vi "gyro_binary_get_time_info.vi"(8 "error in":errorcluster, 10 "all in one package in":T1={"measurement data"={"number of samples per axis"=0, "timestamp array"=[], "offset array"=[], "x, y, z axis data"=[], "magnitude of acceleartion vectors"={"t0"=timestamp(0 s since 1904-01-01), "dt"=1.0, "Y"=[]}, "statistics"={"mean of x axis acceleration"=0.0, "standard devation \nof x axis acceleration"=0.0, "mean of y axis acceleration"=0.0, "standard devation \nof y axis acceleration"=0.0, "mean of z axis acceleration"=0.0, "standard devation \nof z axis acceleration"=0.0, "mean of magnitude\n of acceleration"=0.0, "standard devation \nof magnitude of acceleration"=0.0}, "voltage"={"t0"=timestamp(0 s since 1904-01-01), "dt"=1.0, "Y"=[]}}, "actigraph settings"={"# Pages"=0, "ODR"=0, "xlRange"=0, "gyroRange"=0, "id"=0, "Samplig Freq [Hz]"=0.0, "xlRange in g"=0.0, "gyroRange in dps"=0.0}, "memory structure"={"length of metadata [byte]"=5, "length of page [byte]"=2048, "length of measurement \ndata on page [byte]"=2028, "length of dataset [byte]"=6}, "time informations"={"starting time"=timestamp(0 s since 1904-01-01), "ending time"=timestamp(0 s since 1904-01-01), "dt[s]"=0.0, "sampling rate [Hz]"=0.0, "length"=0.0}} {"time informations"."length" format="%<%H:%M:%S%3u>t"; "actigraph settings"."id" format="%02d"; "actigraph settings"."xlRange" format="%02x"; "actigraph settings"."ODR" format="%02x"}, 11 "pages":u8[](array[numeric])) -> (0 "error out":errorcluster, 2 "all in one package out":T1={"measurement data"={"number of samples per axis"=0, "timestamp array"=[], "offset array"=[], "x, y, z axis data"=[], "magnitude of acceleartion vectors"={"t0"=timestamp(0 s since 1904-01-01), "dt"=1.0, "Y"=[]}, "statistics"={"mean of x axis acceleration"=0.0, "standard devation \nof x axis acceleration"=0.0, "mean of y axis acceleration"=0.0, "standard devation \nof y axis acceleration"=0.0, "mean of z axis acceleration"=0.0, "standard devation \nof z axis acceleration"=0.0, "mean of magnitude\n of acceleration"=0.0, "standard devation \nof magnitude of acceleration"=0.0}, "voltage"={"t0"=timestamp(0 s since 1904-01-01), "dt"=1.0, "Y"=[]}}, "actigraph settings"={"# Pages"=0, "ODR"=0, "xlRange"=0, "gyroRange"=0, "id"=0, "Samplig Freq [Hz]"=0.0, "xlRange in g"=0.0, "gyroRange in dps"=0.0}, "memory structure"={"length of metadata [byte]"=5, "length of page [byte]"=2048, "length of measurement \ndata on page [byte]"=2028, "length of dataset [byte]"=6}, "time informations"={"starting time"=timestamp(0 s since 1904-01-01), "ending time"=timestamp(0 s since 1904-01-01), "dt[s]"=0.0, "sampling rate [Hz]"=0.0, "length"=0.0}} {"time informations"."length" format="%<%H:%M:%S%3u>t"; "actigraph settings"."id" format="%02d"; "actigraph settings"."xlRange" format="%02x"; "actigraph settings"."ODR" format="%02x"}, 3 "pages excluding first and last page":u8[](array[numeric]))   [LabVIEW 2019]
uses:
  Controls/gyro_control_all_in_one_package.ctl
  Controls/gyro_control_measurement_data.ctl
  Controls/gyro_control_measurement_settings.ctl
  Controls/gyro_control_memory_structure.ctl
  Controls/gyro_control_time_informations.ctl
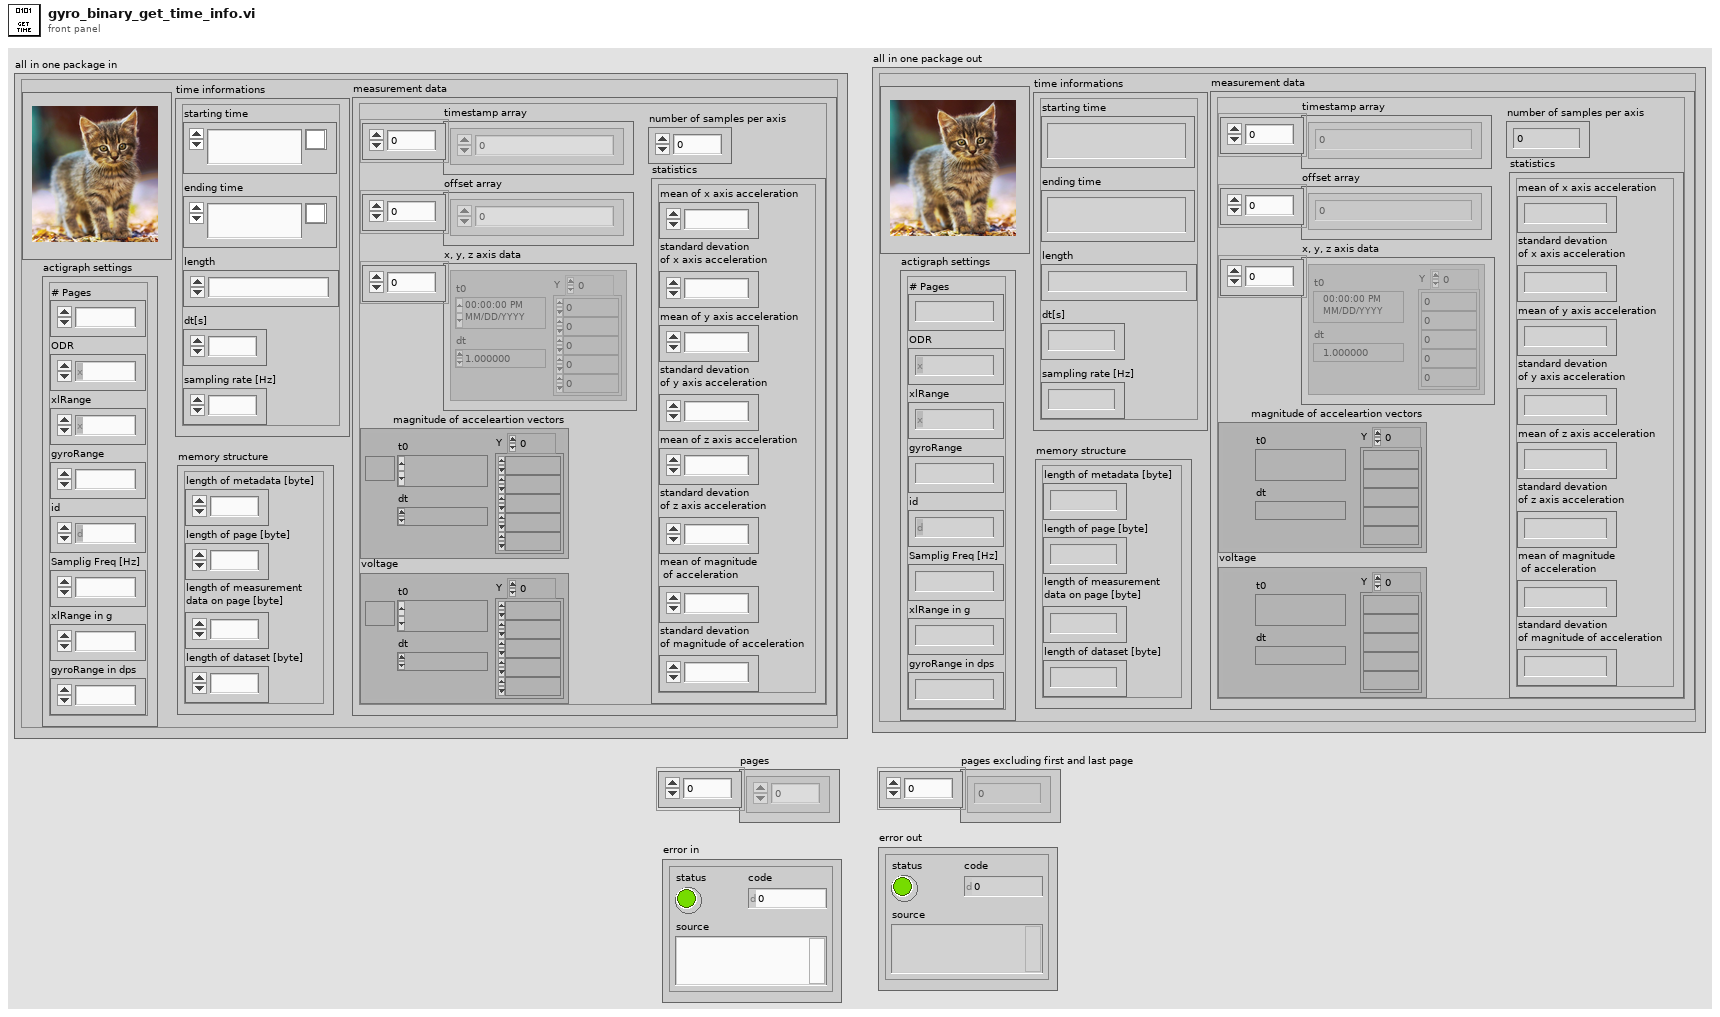
[diagram p1: front panel]
types:
  T1 = typedef "gyro_control_all_in_one_package.ctl" = cluster{"measurement data":T2, "actigraph settings":T3, "memory structure":T4, "time informations":T5}
  T2 = typedef "gyro_control_measurement_data.ctl" = cluster{"number of samples per axis":i32, "timestamp array":dbl[], "offset array":dbl[], "x, y, z axis data":waveform(dbl)[], "magnitude of acceleartion vectors":waveform(dbl), "statistics":cluster{"mean of x axis acceleration":dbl, "standard devation \nof x axis acceleration":dbl, "mean of y axis acceleration":dbl, "standard devation \nof y axis acceleration":dbl, "mean of z axis acceleration":dbl, "standard devation \nof z axis acceleration":dbl, "mean of magnitude\n of acceleration":dbl, "standard devation \nof magnitude of acceleration":dbl}, "voltage":waveform(dbl)}
  T3 = typedef "gyro_control_measurement_settings.ctl" = cluster{"# Pages":i32, "ODR":u8, "xlRange":u8, "gyroRange":u8, "id":u8, "Samplig Freq [Hz]":dbl, "xlRange in g":dbl, "gyroRange in dps":dbl}
  T4 = typedef "gyro_control_memory_structure.ctl" = cluster{"length of metadata [byte]":i32, "length of page [byte]":i32, "length of measurement \ndata on page [byte]":i32, "length of dataset [byte]":i32}
  T5 = typedef "gyro_control_time_informations.ctl" = cluster{"starting time":timestamp, "ending time":timestamp, "dt[s]":dbl, "sampling rate [Hz]":dbl, "length":dbl}
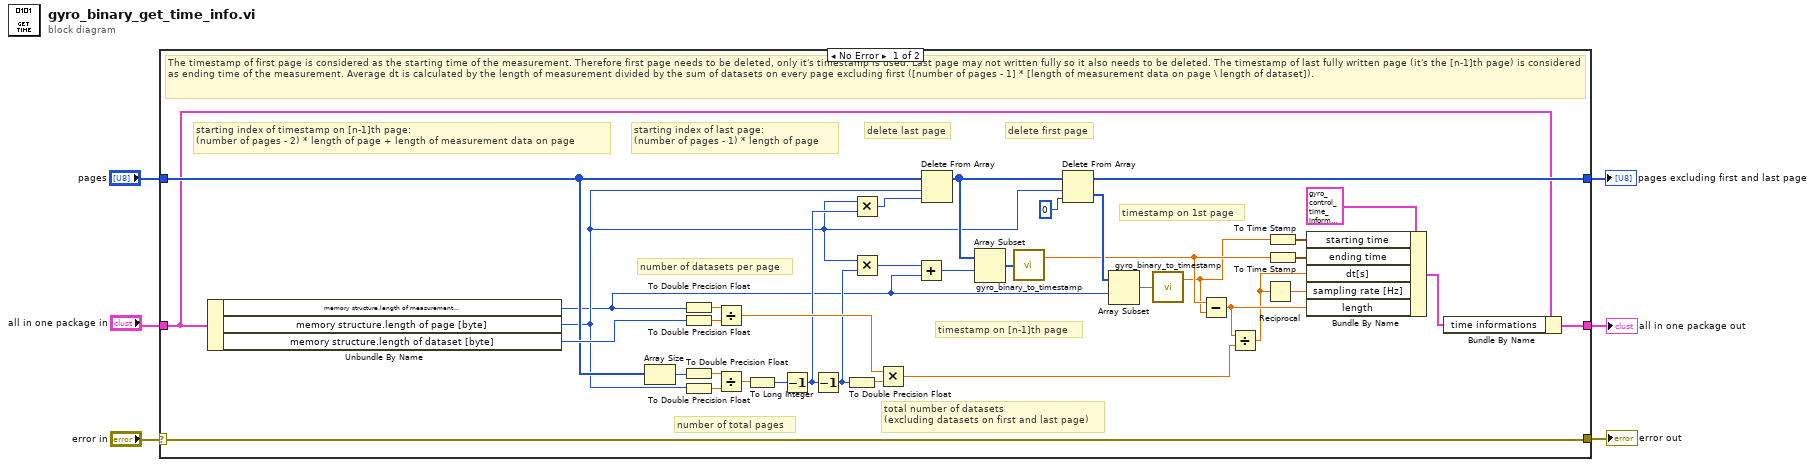
[diagram p0: block diagram]
diagram:
  n1 = case shown="No Error" "error in" {
    selector: "error in" -> [w41 w46]
    tunnel: "pages" -> [w12 w44]
    tunnel: [w41 w46] -> w5
    tunnel: [w15 w44] -> w4
    tunnel: "all in one package in" -> [w11 w45]
    tunnel: [w32 w45] -> w2
    frame No Error {
      # "timestamp on 1st page"
      # "timestamp on [n-1]th page"
      # "starting index of timestamp on [n-1]th page:\n(number of pages - 2) * length of page + length of measurement data on page"
      # "starting index of last page:\n(number of pages - 1) * length of page"
      # "delete first page"
      # "delete last page"
      # "number of total pages"
      # "number of datasets per page"
      # "total number of datasets \n(excluding datasets on first and last page)"
      # "The timestamp of first page is considered as the starting time of the measurement. Therefore first page needs to be deleted, only it's timestamp is used. Last page may not written fully so it also needs to be deleted. The timestamp of last fully written page (it's the [n-1]th page) is considered as ending time of the measurement. Average dt is calculated by the length of measurement divided by the sum of datasets on every page excluding first ([number of pages - 1] * [length of measurement data on page \\ length of dataset])."
      n2 = Unbundle By Name(w11) -> ("memory structure.length of measurement \ndata on page [byte]"=w7:i32, "memory structure.length of page [byte]"=w9:i32, "memory structure.length of dataset [byte]"=w34:i32)
      n3 = Array Size(array=w12) -> (size(s)=w38:i32)
      n4 = To Double Precision Float(number=w7) -> (double precision float=w31:dbl)
      n5 = To Double Precision Float(number=w34) -> (double precision float=w43:dbl)
      n6 = To Double Precision Float(number=w38) -> (double precision float=w37:dbl)
      n7 = To Double Precision Float(number=w9) -> (double precision float=w36:dbl)
      n8 = Divide(x=w31, y=w43) -> (x/y=w42:dbl)
      n9 = Divide(x=w37, y=w36) -> (x/y=w35:dbl)
      n10 = To Long Integer(number=w35) -> (32bit integer=w30:i32)
      n11 = Decrement(x=w30) -> (x-1=w28:i32)
      n12 = Decrement(x=w28) -> (x-1=w13:i32)
      n13 = To Double Precision Float(number=w13) -> (double precision float=w40:dbl)
      n14 = Multiply(x=w9, y=w28) -> (x*y=w29:i32)
      n15 = Multiply(x=w9, y=w13) -> (x*y=w10:i32)
      n16 = Multiply(x=w42, y=w40) -> (x*y=w18:dbl)
      n17 = Add(x=w10, y=w7) -> (x+y=w8:i32)
      n18 = Delete From Array(array=w12, length=w9, index=w29) -> (array with subset deleted=w14:u8[])  [unwired: 1 out]
      n19 = Array Subset(array=w14, index=w8) -> (w25:u8[])  [unwired: 1 in]
      n20 = call "gyro_binary_to_timestamp.vi"("binaryTimestampWithOffset"=w25) -> ("timestamp"=w21:dbl)  [unwired: 1 out]
      n21 = Delete From Array(array=w14, length=w9, index=0) -> (deleted portion=w26:u8[], array with subset deleted=w15:u8[])
      n22 = Array Subset(array=w26, index=w7) -> (w24:u8[])  [unwired: 1 in]
      n23 = call "gyro_binary_to_timestamp.vi"("binaryTimestampWithOffset"=w24) -> ("timestamp"=w20:dbl)  [unwired: 1 out]
      n24 = Subtract(x=w21, y=w20) -> (x-y=w19:dbl)
      n25 = Divide(x=w19, y=w18) -> (x/y=w16:dbl)
      n26 = Reciprocal(x=w16) -> (1/x=w17:dbl)
      n27 = To Time Stamp(1:w20) -> (0:w23:timestamp)
      n28 = To Time Stamp(1:w21) -> (0:w22:timestamp)
      n29 = Bundle By Name(cluster=T5 {"starting time"=timestamp(0 s since 1904-01-01), "ending time"=timestamp(0 s since 1904-01-01), "dt[s]"=0.0, "sampling rate [Hz]"=0.0, "length"=0.0}, "starting time"=w23, "ending time"=w22, "dt[s]"=w16, "sampling rate [Hz]"=w17, "length"=w19) -> (w33:T5)
      n30 = Bundle By Name(cluster=w11, "time informations"=w33) -> (w32:T1)
    }
    frame Error {
    }
  }
  "error out" <- w5
  "pages excluding first and last page" <- w4
  "all in one package out" <- w2
